vi "uService GUI.vi"(8 "error in (no error)":errorcluster, 11 "Error Manager in":refnum<class "Error Manager.lvclass">) -> (3 "Error Manager out":refnum<class "Error Manager.lvclass">)   [LabVIEW 2026, in "TALOS.lvlib" / "Error Manager.lvlib" / "Error Manager.lvclass"]
uses:
  Error Manager.lvclass
  C:/LabVIEW Code/TALOS/talos/Father of all uServices/Father of all uServices/Father of all uServices.lvclass
  Error Info.ctl
  Error Manager.lvclass/Error Manager.ctl
  Ancestor/Ancestor/Ancestor.lvclass/Ancestor.ctl
  Read Distributed flag.vi
  Support VIs/Substitute Error.vi
  Support VIs/Generate Error.vi
  FGV/Error Memory/Get Error Description.vi
  Support VIs/Get PC name.vi
  Ancestor/Ancestor/Read ID.vi
  Support VIs/Get Class Name.vi
  FGV/Error Memory/Error Memory Core.vi
  <vilib>/AdvancedString/Delimited String to 1D String Array.vi
  <vilib>/AdvancedString/Delimited String to 1D String Array (string).vi
  Support VIs/Circus Root Path.vi
  FGV/Error Memory/Error Crt Lvl checker.vi
  FGV/Error Memory/Error Memory Core.vi/40c8088d-b597-4017-91af-faa98e00292e.vi
  FGV/Error Memory/Error Memory Core.vi/d4a3ab98-063c-4e44-b43d-fbdcfe6c2be2.vi
  Father of all uServices/Father of all uServices/Father of all uServices.lvclass
  C:/LabVIEW Code/TALOS/builds/Actor Framework PPL/Actor Framework.lvlibp/1abvi3w/vi.lib/ActorFramework/Actor/Actor.lvclass
  Support VIs/Global Memory.vi
  builds/Actor Framework PPL/Actor Framework.lvlibp/1abvi3w/vi.lib/ActorFramework/Actor/Read Self Enqueuer.vi
  builds/Actor Framework PPL/Actor Framework.lvlibp/1abvi3w/vi.lib/ActorFramework/Stop Msg/Send Normal Stop.vi
  <vilib>/Utility/LVClass/Get LV Class Name.vi
  Support VIs/Is in Packed Library.vi
  Support VIs/TALOS Root path.vi
  Support VIs/Read CSV worksheet.vi
  Support VIs/Global Constants.vi
  <vilib>/Utility/error.llb/General Error Handler.vi
  Support VIs/Error Log.vi
  Ancestor/Ancestor/Ancestor.lvclass
  <vilib>/Comparison/Equal/Equal Functor/Equal Functor.lvclass
  TALOS.lvlib
panel:
  out "Distributed Error Manager online":bool
  out "INFO":string="Local Error Manager propagates error from the Guardian to the Distributed Error Manager (aka Error Manager). If the Distributed Error Manager isn't available, the Local Error Manager will display errors instead.\nThe Local Error Manager also filters errors on the Guardian."
  in  "Clear Filters":bool
  in  "Filter out Errors":bool
  in  "Errors to filter":i32[](array[numeric])
  in  "Suppress error pop-ups":bool
  in  "Dismiss All Errors":bool
  in  "Generate Error":bool
  in  "Error to generate":errorcluster
  in  "Dismiss Errror":bool
  out "Error Details Display":string
  in  "View Error Details":bool
  in  "Select Error":i32 min=0
  out "Array of Errors Display":T1[](array[typedef]) {"Time Stamp" format="%<%x %.3X>T"}
  in  "stop New uService":bool
  out "ID":string="Error Manager"
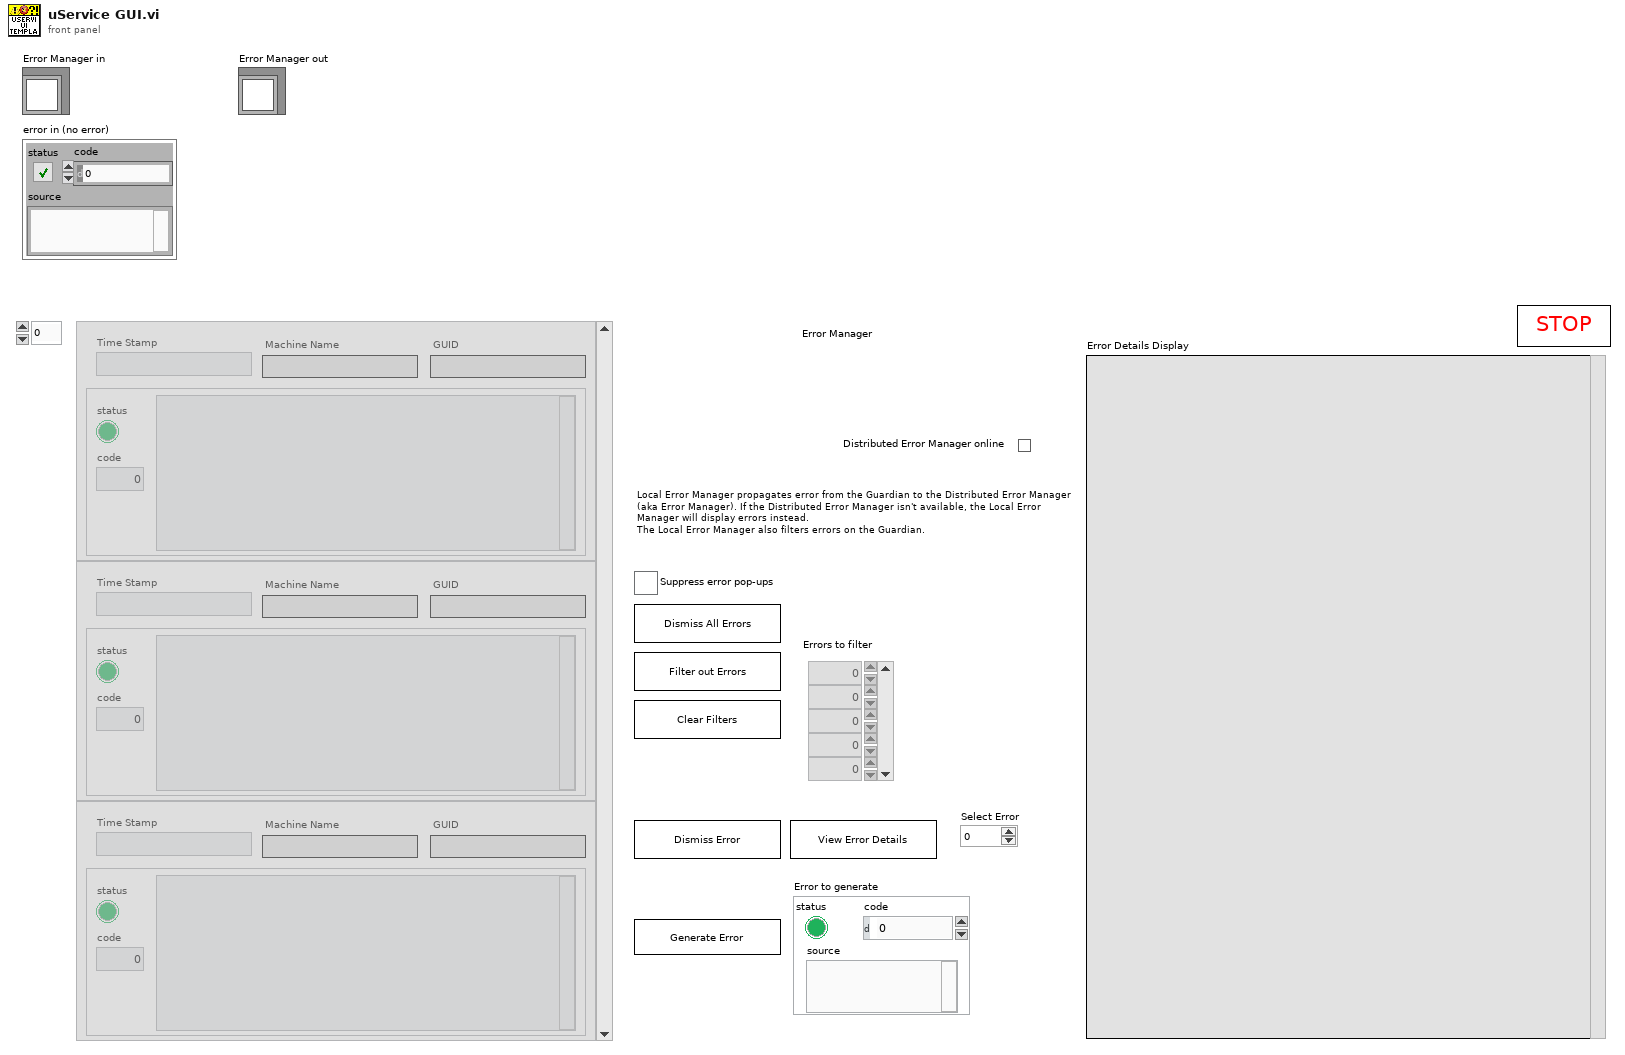
[diagram p1: front panel]
types:
  T1 = typedef "TALOS.lvlib/Error Manager.lvlib/Error Manager.lvclass/Error Info.ctl" = cluster{"error out":errorcluster, "Time Stamp":timestamp, "Machine Name":string, "GUID":string}
  T2 = enum8{"Enabled", "Disabled", "Disabled and Grayed Out"}
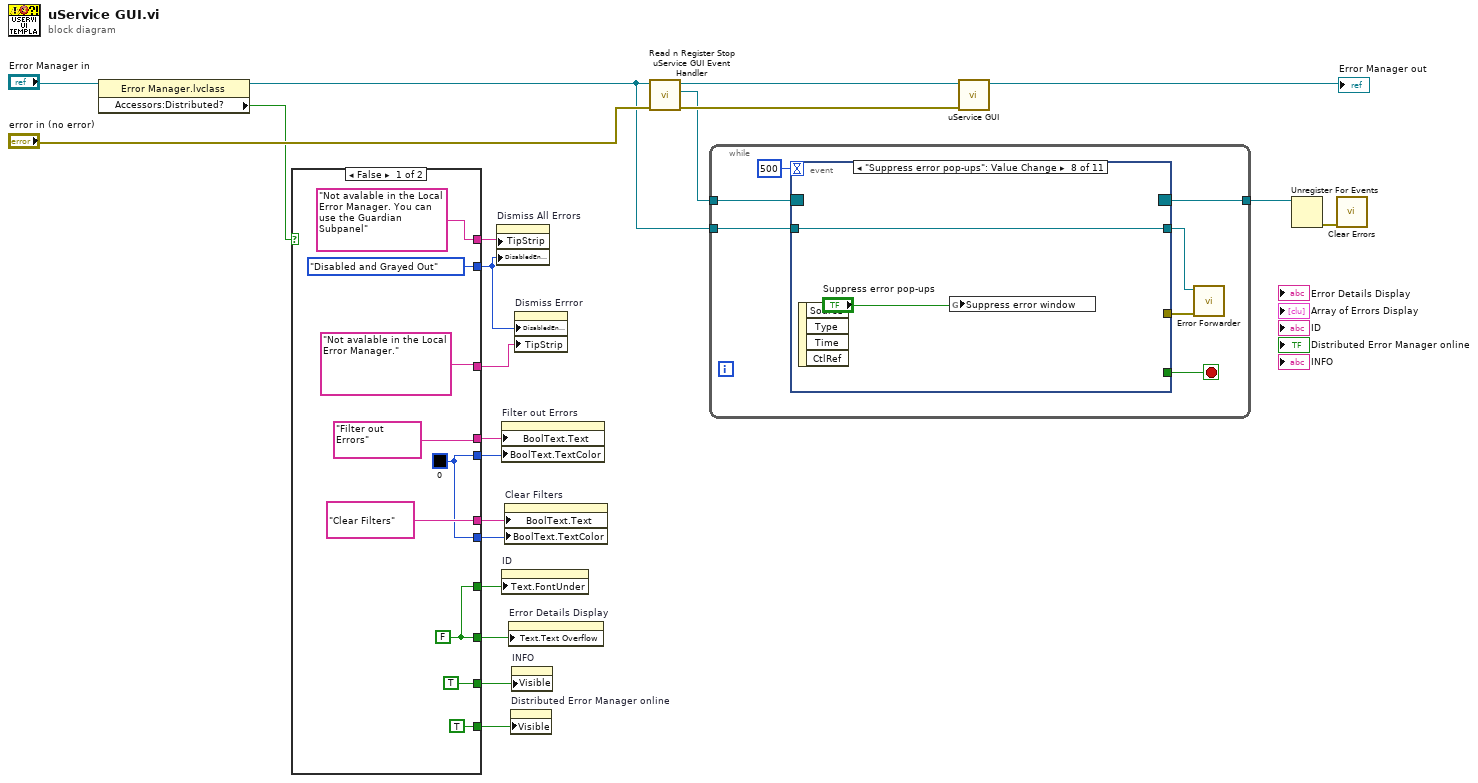
[diagram p0: block diagram]
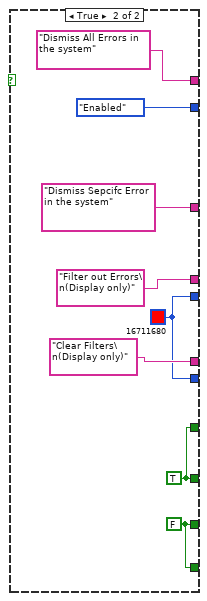
[diagram p2: hidden frame]
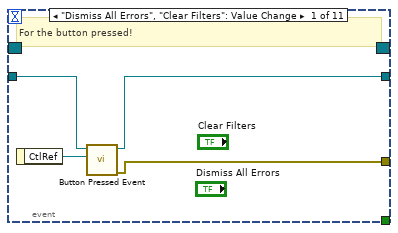
[diagram p3: hidden frame]
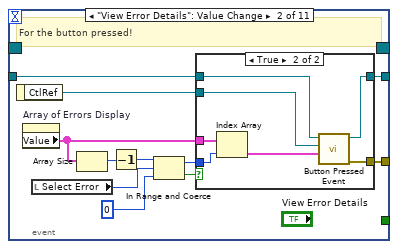
[diagram p4: hidden frame]
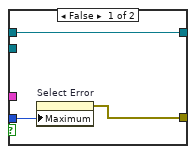
[diagram p5: hidden frame]
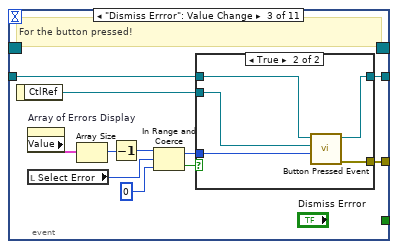
[diagram p6: hidden frame]
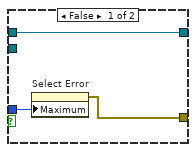
[diagram p7: hidden frame]
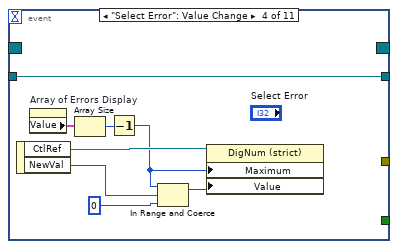
[diagram p8: hidden frame]
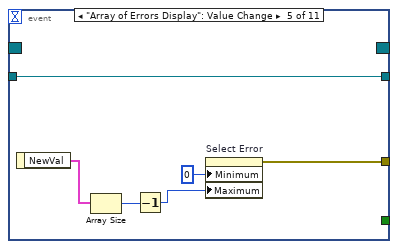
[diagram p9: hidden frame]
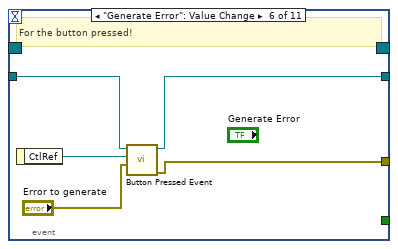
[diagram p10: hidden frame]
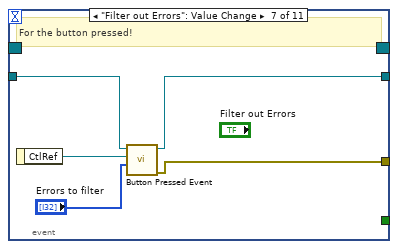
[diagram p11: hidden frame]
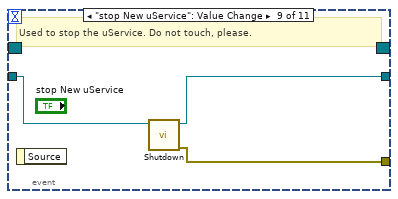
[diagram p12: hidden frame]
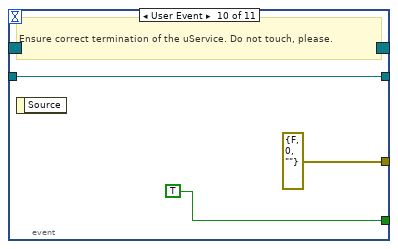
[diagram p13: hidden frame]
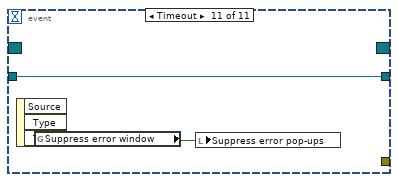
[diagram p14: hidden frame]
diagram:
  n1 = property class="Error Manager.lvclass"(reference="Error Manager in") -> (reference out=w13:refnum<class "Error Manager.lvclass">, "Accessors:Distributed?"=w12:bool)  [unwired: 1 in, 1 out]
  n2 = case shown="False" w12 {
    tunnel: [T2."Disabled and Grayed Out" ("Disabled") T2."Enabled" ("Disabled")] -> w10
    tunnel: ["Not avalable in the Local Error Manager. You can use the Guardian Subpanel" ("Tip Strip") "Dismiss All Errors in the system" ("Tip Strip")] -> w11
    tunnel: ["Not avalable in the Local Error Manager." ("Tip Strip") "Dismiss Sepcifc Error in the system" ("Tip Strip")] -> w9
    tunnel: ["Filter out Errors" ("Boolean Text.Text") "Filter out Errors\n(Display only)" ("Boolean Text.Text")] -> w8
    tunnel: ["Clear Filters" ("Boolean Text.Text") "Clear Filters\n(Display only)" ("Boolean Text.Text")] -> w7
    tunnel: [w25 w33] -> w6
    tunnel: [w25 w33] -> w5
    tunnel: [w24 w32] -> w4
    tunnel: [w24 w32] -> w3
    tunnel: [TRUE ("Visible") w31] -> w2
    tunnel: [TRUE ("Visible") w31] -> w1
    frame False {
      w24 = FALSE ("Text.Text Overflow")
      w25 = u32 0 ("Boolean Text.Text Colors:Text Color")
    }
    frame True {
      w31 = FALSE ("Visible")
      w32 = TRUE ("Text.Text Overflow")
      w33 = u32 16711680 ("Boolean Text.Text Colors:Text Color")
    }
  }
  n3 = property on="Dismiss All Errors" class="Bool"("TipStrip"=w11, "DisabledEnum"=w10) -> ()  [unwired: 2 in, 2 out]
  n4 = property on="Filter out Errors" class="Bool"("BoolText.Text"=w8, "BoolText.TextColor"=w6) -> ()  [unwired: 2 in, 2 out]
  n5 = property on="ID" class="Str"("Text.FontUnder"=w4) -> ()  [unwired: 2 in, 2 out]
  n6 = property on="Clear Filters" class="Bool"("BoolText.Text"=w7, "BoolText.TextColor"=w5) -> ()  [unwired: 2 in, 2 out]
  n7 = property on="Error Details Display" class="Str"("Text.Text Overflow"=w3) -> ()  [unwired: 2 in, 2 out]
  n8 = property on="Distributed Error Manager online" class="Bool (strict)"("Visible"=w1) -> ()  [unwired: 2 in, 2 out]
  n9 = property on="INFO" class="Str"("Visible"=w2) -> ()  [unwired: 2 in, 2 out]
  n10 = property on="Dismiss Errror" class="Bool"("DisabledEnum"=w10, "TipStrip"=w9) -> ()  [unwired: 2 in, 2 out]
  n11 = call-dynamic "Read n Register Stop uService GUI Event Handler .vi"("error in (no error)"="error in (no error)", "uService Template in"=w13) -> ("error out"=w19:errorcluster, "Stop uService GUI Event Ref"=w18:refnum<event-registration>, "uService Template out"=w20:refnum<class "Error Manager.lvclass">)  [unwired: 7 in]
  n12 = while {
    tunnel: [w45] -> w21
    tunnel: w18 -> [w43]
    tunnel: w13 -> [w42]
    stop <- w44 stop-if-true
    n13 = event shown="[7] \"Suppress error pop-ups\": Value Change" {
      selector: w43 -> [_ _ _ _ _ _ _ _ _ _ _]
      dyn-events: [_ _ _ _ _ _ _ _ _ _ _] -> w45
      timeout: 500 -> [_ _ _ _ _ _ _ _ _ _ _]
      tunnel: [_ _ _ _ _ _ _ _ _ TRUE _] -> w44
      tunnel: w42 -> [w49 w60 w81 w90 w98 w108 w113 w114 w118 w120 w123]
      tunnel: [w47 w55 w75 w90 w98 w106 w111 w114 w117 w120 w123] -> w40
      tunnel: [w46 w58 w79 _ w103 w105 w110 _ w116 errorcluster {"status"=FALSE, "code"=0, "source"=""} ("error in (no error)") _] -> w41
      event "Dismiss All Errors", "Clear Filters": Value Change {
        # "For the button pressed!"
        n14 = event-data() -> ("CtlRef"=w48:refnum<vi>)  [unwired: 1 in]
        n15 = call-dynamic "Button Pressed Event.vi"("CtlRef"=w48, "uService Template in"=w49) -> ("error out"=w46:errorcluster, "uService Template out"=w47:refnum<class "Error Manager.lvclass">)  [unwired: 8 in]
      }
      event "View Error Details": Value Change {
        # "For the button pressed!"
        n16 = event-data() -> ("CtlRef"=w59:refnum<vi>)  [unwired: 1 in]
        n17 = property on="Array of Errors Display" class="Arr (strict)"() -> ("Value"=w51:T1[])  [unwired: 2 in, 2 out]
        n18 = local read "Select Error"() -> (w50:i32)
        n19 = Array Size(array=w51) -> (size(s)=w54:i32)
        n20 = Decrement(x=w54) -> (x-1=w53:i32)
        n21 = In Range and Coerce(upper limit=w53, x=w50, lower limit=0) -> (coerced(x)=w52:i32, In Range?=w56:bool)
        n22 = case shown="True" w56 {
          tunnel: w60 -> [w63 w68]
          tunnel: w59 -> [_ w70]
          tunnel: [w62 w69] -> w58
          tunnel: [w63 w67] -> w55
          tunnel: w52 -> [w61 w66]
          tunnel: w51 -> [_ w65]
          frame False {
            n23 = property on="Select Error" class="DigNum (strict)"("Maximum"=w61) -> (error out=w62:errorcluster)  [unwired: 2 in, 1 out]
          }
          frame True {
            n24 = Index Array(array=w65, index=w66) -> (element=w64:T1)
            n25 = call-dynamic "Button Pressed Event.vi"("Data"=w64, "CtlRef"=w70, "uService Template in"=w68) -> ("error out"=w69:errorcluster, "uService Template out"=w67:refnum<class "Error Manager.lvclass">)  [unwired: 7 in]
          }
        }
      }
      event "Dismiss Errror": Value Change {
        # "For the button pressed!"
        n26 = event-data() -> ("CtlRef"=w80:refnum<vi>)  [unwired: 1 in]
        n27 = property on="Array of Errors Display" class="Arr (strict)"() -> ("Value"=w78:T1[])  [unwired: 2 in, 2 out]
        n28 = local read "Select Error"() -> (w71:i32)
        n29 = Array Size(array=w78) -> (size(s)=w74:i32)
        n30 = Decrement(x=w74) -> (x-1=w73:i32)
        n31 = In Range and Coerce(upper limit=w73, x=w71, lower limit=0) -> (coerced(x)=w72:i32, In Range?=w76:bool)
        n32 = case shown="True" w76 {
          tunnel: w81 -> [w84 w87]
          tunnel: w80 -> [_ w89]
          tunnel: [w82 w88] -> w79
          tunnel: [w84 w86] -> w75
          tunnel: w72 -> [w83 w85]
          frame False {
            n33 = property on="Select Error" class="DigNum (strict)"("Maximum"=w83) -> (error out=w82:errorcluster)  [unwired: 2 in, 1 out]
          }
          frame True {
            n34 = call-dynamic "Button Pressed Event.vi"("Data"=w85, "CtlRef"=w89, "uService Template in"=w87) -> ("error out"=w88:errorcluster, "uService Template out"=w86:refnum<class "Error Manager.lvclass">)  [unwired: 7 in]
          }
        }
      }
      event "Select Error": Value Change {
        n35 = event-data() -> ("CtlRef"=w97:refnum<vi>, "NewVal"=w92:i32)  [unwired: 1 in]
        n36 = property on="Array of Errors Display" class="Arr (strict)"() -> ("Value"=w96:T1[])  [unwired: 2 in, 2 out]
        n37 = Array Size(array=w96) -> (size(s)=w95:i32)
        n38 = Decrement(x=w95) -> (x-1=w94:i32)
        n39 = In Range and Coerce(upper limit=w94, x=w92, lower limit=u32 0) -> (coerced(x)=w91:u32)  [unwired: 1 out]
        n40 = property class="DigNum (strict)"(reference=w97, "Maximum"=w94, "Value"=w91) -> ()  [unwired: 1 in, 2 out]
      }
      event "Array of Errors Display": Value Change {
        n41 = event-data() -> ("NewVal"=w102:T1[])  [unwired: 1 in]
        n42 = Array Size(array=w102) -> (size(s)=w101:i32)
        n43 = Decrement(x=w101) -> (x-1=w99:i32)
        n44 = property on="Select Error" class="DigNum (strict)"("Minimum"=0 ("Data Entry Limits:Minimum"), "Maximum"=w99) -> (error out=w103:errorcluster)  [unwired: 2 in, 1 out]
      }
      event "Generate Error": Value Change {
        # "For the button pressed!"
        n45 = event-data() -> ("CtlRef"=w107:refnum<vi>)  [unwired: 1 in]
        n46 = call-dynamic "Button Pressed Event.vi"("Data"="Error to generate", "CtlRef"=w107, "uService Template in"=w108) -> ("error out"=w105:errorcluster, "uService Template out"=w106:refnum<class "Error Manager.lvclass">)  [unwired: 7 in]
      }
      event "Filter out Errors": Value Change {
        # "For the button pressed!"
        n47 = event-data() -> ("CtlRef"=w112:refnum<vi>)  [unwired: 1 in]
        n48 = call-dynamic "Button Pressed Event.vi"("Data"="Errors to filter", "CtlRef"=w112, "uService Template in"=w113) -> ("error out"=w110:errorcluster, "uService Template out"=w111:refnum<class "Error Manager.lvclass">)  [unwired: 7 in]
      }
      event "Suppress error pop-ups": Value Change {
        n49 = event-data() -> ()  [unwired: 1 in, 4 out]
        n50 = global write "Global Memory.vi" "Suppress error window"("Suppress error pop-ups") -> ()
      }
      event "stop New uService": Value Change {
        # "Used to stop the uService. Do not touch, please."
        n51 = event-data() -> ()  [unwired: 1 in, 1 out]
        n52 = call "Shutdown.vi"("Father of all uServices in"=w118) -> ("error out"=w116:errorcluster, "Father of all uServices out"=w117:refnum<class "Error Manager.lvclass">)  [unwired: 9 in]
      }
      event User Event {
        # "Ensure correct termination of the uService. Do not touch, please."
        n53 = event-data() -> ()  [unwired: 1 in, 1 out]
      }
      event Timeout {
        n54 = event-data() -> ()  [unwired: 1 in, 3 out]
        n55 = global read "Global Memory.vi" "Suppress error window"() -> (w122:bool)
        n56 = local write "Suppress error pop-ups"(w122) -> ()
      }
    }
    n57 = call "Error Forwarder.vi"("error in (no error)"=w41, "Father of all uServices in"=w40) -> ()  [unwired: 10 in]
  }
  n58 = call-parent "uService GUI.vi"("error in (no error)"=w19, "uService Template in"=w20) -> ("uService Template out"=→"Error Manager out":refnum<class "Error Manager.lvclass">)  [unwired: 9 in]
  n59 = Unregister For Events(event registration refnum=w21) -> (error out=w14:errorcluster)  [unwired: 1 in]
  n60 = call <vilib>:"Clear Errors.vi"("error in (no error)"=w14) -> ()  [unwired: 5 in, 2 out]
